vi "GetNodeName.vi"(0 "reference in":refnum<class "VINode.lvclass">, 5 "error in (no error)":errorcluster) -> (14 "reference out":refnum<class "VINode.lvclass">, 15 "String":string, 19 "error out":errorcluster)   [LabVIEW 2014, in "VINode.lvclass"]
uses:
  <resource>/Framework/Providers/Open_GDS/UML/VINode_class/VINode.lvclass
  <resource>/Framework/Providers/Open_GDS/UML/MultiLineString_class/MultiLineString.lvclass
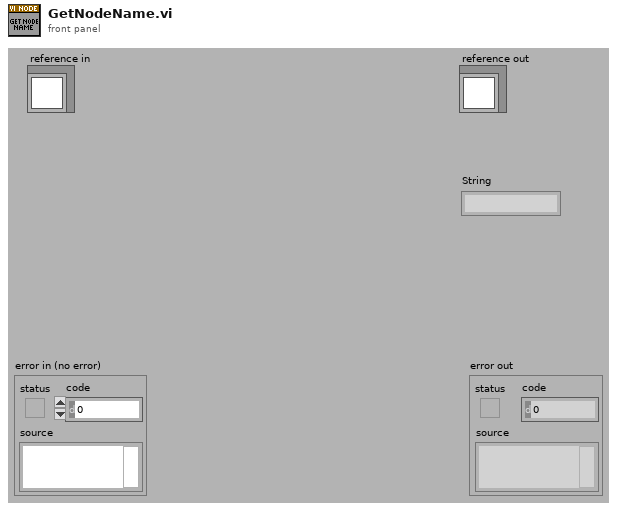
[diagram p1: front panel]
types:
  T1 = typedef "VINode.lvclass/ObjectAttributes.ctl" = cluster{"midHeight":dbl, "botHeight":dbl, "Name":refnum<class "MultiLineString.lvclass">, "DEFAULT_COMPARTMENT_HEIGHT":i32, "DEFAULT_WIDTH":i32, "DEFAULT_HEIGHT":i32, "VIPath":path, "Description":refnum<class "MultiLineString.lvclass">, "ShowDescription":bool}
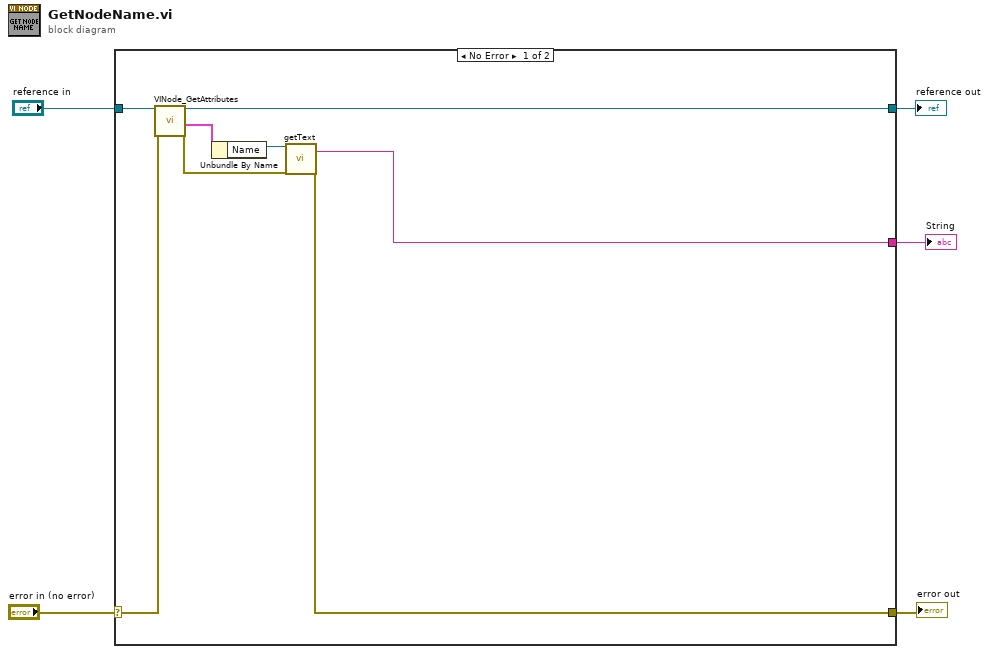
[diagram p0: block diagram]
diagram:
  n1 = case shown="No Error" "error in (no error)" {
    selector: "error in (no error)" -> [w13 w15]
    tunnel: [w8 w15] -> w4
    tunnel: [w11 w14] -> w2
    tunnel: "reference in" -> [w12 w14]
    tunnel: [w7 _] -> w1
    frame No Error {
      n2 = call <resource>:"VINode_GetAttributes.vi"("reference in"=w12, "error in (no error)"=w13) -> ("reference out"=w11:refnum<class "VINode.lvclass">, "Data"=w6:T1, "error out"=w9:errorcluster)  [unwired: 14 in, 1 out]
      n3 = Unbundle By Name(w6) -> ("Name"=w10:refnum<class "MultiLineString.lvclass">)
      n4 = call-dynamic "getText.vi"("reference"=w10, "error in (no error)"=w9) -> ("text"=w7:string, "error out"=w8:errorcluster)  [unwired: 15 in, 1 out]
    }
    frame Error {
    }
  }
  "error out" <- w4
  "reference out" <- w2
  "String" <- w1
